vi "Reserve AI.vi"(8 "error in (no error)":errorcluster, 9 "Purpose":string, 10 "ADC #":T1=-1, 11 "Session in":refnum<class "Session.lvclass">) -> (0 "error out":errorcluster, 3 "Session out":refnum<class "Session.lvclass">)   [LabVIEW 2024, in "CTI.lvlib" / "Session.lvclass"]
uses:
  Session.lvclass
  ADC Number.ctl
  AI/AI.lvclass/AI.ctl
  GPIO/GPIO.lvclass/GPIO.ctl
  Session.lvclass/Session.ctl
  4ea076bf-f3e9-4c16-b6f7-46e9efeaade7.vi
  aa173da3-1a13-4d27-92e2-a587cb8a43f6.vi
  aa173da3-1a13-4d27-92e2-a587cb8a43f6.vi/685f7f19-b444-4620-8f66-e6e2ddd64bb8.vi
  AI/AI.lvclass
  C:/Users/nkirchne/Documents/~SANDBOX/Electronics Workflow/build/ForPort/CTI/Resource/Resource.lvclass
  Generate Error.vi
  Resource/Resource.lvclass
  CTI.lvlib
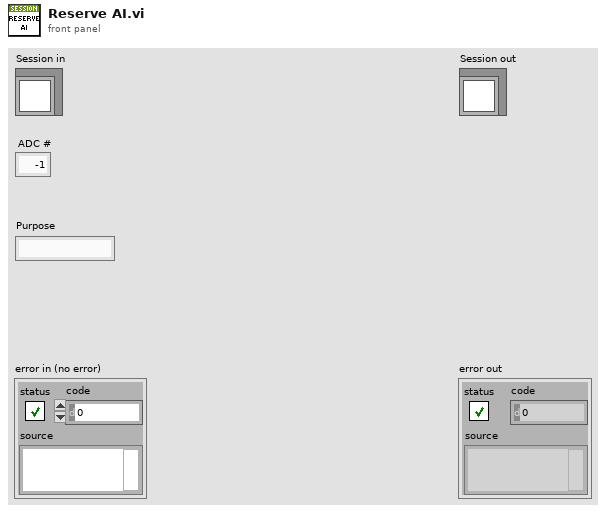
[diagram p1: front panel]
types:
  T1 = typedef "CTI.lvlib/ADC Number.ctl" = i8
  T2 = typedef "CTI.lvlib/GPIO Number.ctl" = i8
  T3 = typedef "CTI.lvlib/Session.lvclass/Resources.ctl" = cluster{"GPIO":map{T2, refnum<class "GPIO.lvclass">}, "AI":map{T1, refnum<class "AI.lvclass">}, "PWM":map{T2, refnum<class "PWM.lvclass">}, "UART":map{T4, refnum<class "UART.lvclass">}, "I2C":map{T5, refnum<class "I2C.lvclass">}, "SPI":map{T6, refnum<class "SPI.lvclass">}, "SPI CS":map{T2, refnum<class "SPI CS.lvclass">}}
  T4 = typedef "CTI.lvlib/UART Number.ctl" = i8
  T5 = typedef "CTI.lvlib/I2C Number.ctl" = i8
  T6 = typedef "CTI.lvlib/SPI Number.ctl" = i8
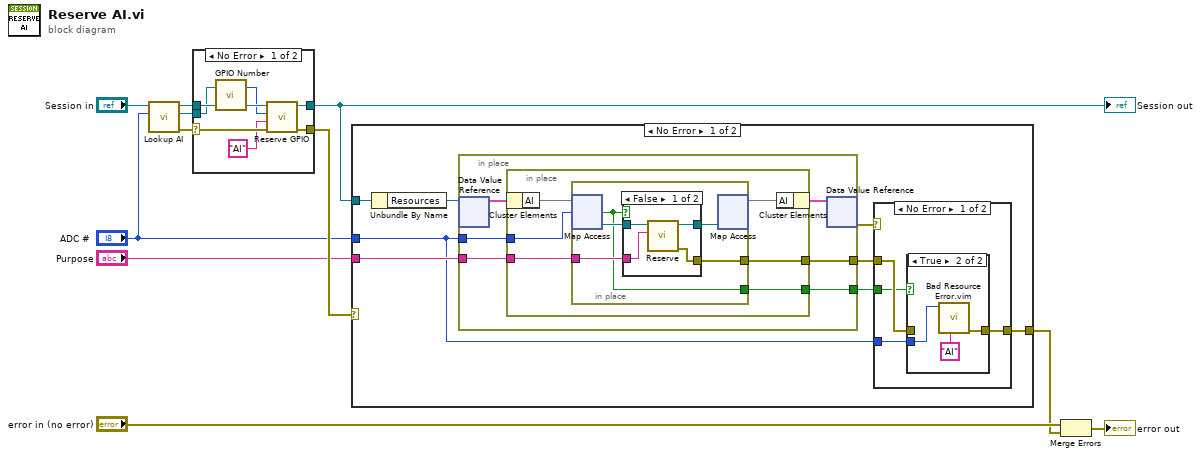
[diagram p0: block diagram]
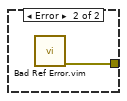
[diagram p4: hidden frame]
diagram:
  n1 = call "Lookup AI.vi"("ADC #"="ADC #", "Session in"="Session in") -> ("error out"=w10:errorcluster, "AI"=w2:refnum<class "AI.lvclass">, "Session out"=w4:refnum<class "Session.lvclass">)  [unwired: 7 in]
  n2 = case shown="No Error" w10 {
    selector: w10 -> [w17 w20]
    tunnel: [w18 w20] -> w11
    tunnel: w4 -> [w16 w19]
    tunnel: w2 -> [w15 _]
    tunnel: [w14 w19] -> w1
    frame No Error {
      n3 = call "GPIO Number.vi"("AI in"=w15) -> ("GPIO #"=w13:T2)  [unwired: 6 in]
      n4 = call "Reserve GPIO.vi"("error in (no error)"=w17, "Purpose"="AI", "GPIO #"=w13, "Session in"=w16) -> ("error out"=w18:errorcluster, "Session out"=w14:refnum<class "Session.lvclass">)  [unwired: 6 in]
    }
    frame Error {
    }
  }
  "Session out" <- w1
  n5 = case shown="No Error" w11 {
    selector: w11 -> [_ w60]
    tunnel: "Purpose" -> [w27 _]
    tunnel: [w23 w60] -> w5
    tunnel: "ADC #" -> [w22 _]
    tunnel: w1 -> [w21 _]
    frame No Error {
      n6 = Unbundle By Name(w21) -> ("Resources"=w28:refnum<data-value>)
      n7 = in-place {
        in-place-border: w22 -> [w43]
        in-place-border: w27 -> [w42]
        in-place-border: [w41] -> w24
        in-place-border: [w40] -> w26
        n8 = in-place-dvr #1(w28) -> (w38:T3)  [unwired: 1 out]
        n9 = in-place {
          in-place-border: w43 -> [w48]
          in-place-border: w42 -> [w47]
          in-place-border: [w46] -> w41
          in-place-border: [w45] -> w40
          n10 = in-place-cluster #2(w38) -> ("AI"=w49:map{T1, refnum<class "AI.lvclass">})
          n11 = in-place {
            in-place-border: w47 -> [w53]
            in-place-border: [w52] -> w45
            in-place-border: [w51] -> w46
            n12 = in-place-map #3(w49, w48) -> (w54:refnum<class "AI.lvclass">, w51:bool)  [unwired: 1 in]
            n13 = case shown="False" w51 {
              tunnel: w54 -> [w58 w59]
              tunnel: w53 -> [w57 _]
              tunnel: [w56 w59] -> w50
              tunnel: [w55 _] -> w52
              frame False {
                n14 = call "Reserve.vi"("Purpose"=w57, "Resource in"=w58) -> ("error out"=w55:errorcluster, "Resource out"=w56:refnum<class "AI.lvclass">)  [unwired: 8 in]
              }
              frame True {
              }
            }
            n15 = in-place-map #3(w50) -> (w44:map{T1, refnum<class "AI.lvclass">})  [unwired: 1 in, 2 out]
          }
          n16 = in-place-cluster #2("AI"=w44) -> (w39:T3)
        }
        n17 = in-place-dvr #1(w39) -> (w25:errorcluster)  [unwired: 1 out]
      }
      n18 = case shown="No Error" w25 {
        tunnel: w26 -> [w32 _]
        tunnel: w24 -> [w31 _]
        tunnel: [w30 w37] -> w23
        tunnel: w22 -> [w29 _]
        frame No Error {
          n19 = case shown="True" w31 {
            tunnel: w32 -> [w33 _]
            tunnel: [w33 w36] -> w30
            tunnel: w29 -> [_ w35]
            frame False {
            }
            frame True {
              n20 = call "Bad Resource Error.vim"("Resource Type"="AI", "Res #"=w35) -> ("error out"=w36:errorcluster)  [unwired: 9 in]
            }
          }
        }
        frame Error {
          n21 = call "Bad Ref Error.vim"() -> ("error out"=w37:errorcluster)  [unwired: 10 in, 1 out]
        }
      }
    }
    frame Error {
    }
  }
  n22 = Merge Errors("error in (no error)", w5) -> (→"error out":errorcluster)
